vi "Remove All Endpoints.vi"(8 "error in (no error)":errorcluster, 11 "Endpoint Config Section Ref in":T1 format="%.0x") -> (0 "error out":errorcluster, 1 "Removed":bool, 3 "Endpoint Config Section Ref out":T1 format="%.0x")   [LabVIEW 2017, in "SLSC Switch Scripting.lvlib"]
uses:
  SLSC Switch Scripting.lvlib
  <vilib>/NI Veristand/Custom Device API/Custom Device Item Ref.ctl
  <vilib>/NI VeriStand/Custom Device API/Custom Device API.lvlib
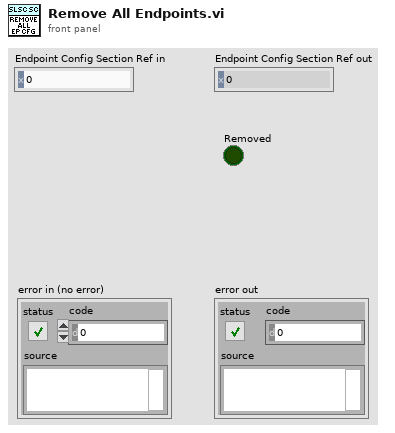
[diagram p1: front panel]
types:
  T1 = typedef "Custom Device API.lvlib/Custom Device Item Ref.ctl" = u64
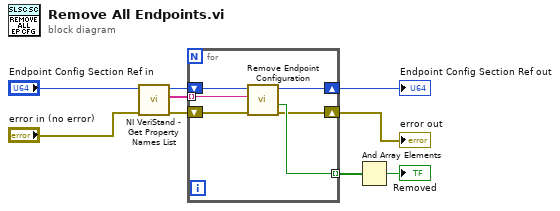
[diagram p0: block diagram]
diagram:
  n1 = call <vilib>:"NI VeriStand - Get Property Names List.vi"("error in (no error)"="error in (no error)", "Item Ref in"="Endpoint Config Section Ref in") -> ("error out"=w8:errorcluster, "Property Names"=w9:string[], "Item Ref out"=w4:T1)  [unwired: 7 in]
  n2 = for {
    tunnel: w9 -> [w13] mode=indexing
    shift-right: [w10] -> w6
    shift-left: w8 -> [w12]
    shift-right: [w14] -> w3
    shift-left: w4 -> [w15]
    tunnel: [w11] -> w1 mode=indexing
    n3 = call "Remove Endpoint Configuration.vi"("error in (no error)"=w12, "Endpoint"=w13, "Endpoint Config Section Ref in"=w15) -> ("error out"=w10:errorcluster, "Removed"=w11:bool, "Endpoint Config Section Ref out"=w14:T1)  [unwired: 6 in]
  }
  "error out" <- w6
  "Endpoint Config Section Ref out" <- w3
  n4 = And Array Elements(Boolean array=w1) -> (logical AND=→"Removed":bool)
